vi "svfa_Process FRF (Nx1).vi"(0 "stimulus signal X [EUx]":waveform(dbl), 1 "response signals Y [EUy]":waveform(dbl)[](array[waveform]), 2 "window":T9=1 items=["None"=0, "Hanning"=1, "Hamming"=2, "Blackman-Harris"=3, "Exact Blackman"=4, "Blackman"=5, "Flat Top"=6, "4 Term B-Harris "=7, "7 Term B-Harris"=8, "Low Sidelobe"=9, "Force - Exponential"=10, "Blackman Nuttall"=11, "Triangle"=30, "Bartlett-Hanning"=31, "Bohman"=32, "Parzen"=33, "Welch"=34, "Kaiser"=60, "Dolph-Chebyshev"=61, "Gaussian"=62], 3 "force/exp settings":T8={"force window [%]"=50.0, "exp window [%]"=10.0} {"exp window [%]" min=0.0 max=100.0 format="%.2f"; "force window [%]" min=0.0 max=100.0 format="%.2f"}, 4 "averaging parameters":T11={"averaging mode"=enum."No averaging", "weighting mode"=enum."Linear", "number of averages"=10, "linear mode"=enum."Auto restart"}, 5 "error in (no error)":errorcluster, 7 "processing control":T10(ring), 9 "FRF mode":enum16{"H1", "H2", "H3"}(ring), 11 "spectra info in":T1[](array[typedef]) {"x-axis units" items=["Time (s)"=0, "Frequency-CB (Hz)"=1, "Frequency-CPB (Hz)"=1248, "Frequency-Arbitrary (Hz)"=2357, "Quefrency (s)"=2, "Revolutions (rev)"=3, "Order"=4, "Speed (RPM)"=11, "Speed (rad/s)"=21, "Index"=65535]; "weighting filter" items=["Linear", "A-weighting", "B-weighting", "C-weighting", "ITU-R 468-4", "Dolby", "CCITT", "C-message", "Wb", "Wc", "Wd", "We", "Wf", "Wh", "Wj", "Wk", "Wm", "AES17 20 kHz lowpass", "AES17 40 kHz lowpass", "AES17 20 kHz highpass", "AES17 40 kHz highpass"]; "dB reference [EU]" format="%.2f"; "engineering units" items=["custom..."=0, "V"=1, "A"=21, "C"=30, "pC"=31, "s"=32, "-"=29, "Pa"=2, "N"=20, "g"=3, "m/s^2"=4, "m/s"=5, "m"=6, "mm/s"=12, "mm"=13, "micron/s"=14, "micron"=15, "in/s^2"=7, "in/s"=8, "in"=9, "mil/s"=10, "mil"=11, "rad/s^2"=16, "rad/s"=17, "rad"=18, "deg/s^2"=26, "deg/s"=27, "deg"=28, "RPM"=22, "cycle/s^2"=23, "Hz"=24, "cycle"=25, "strain"=19]; "spectral info"."window" items=["None "=0, "Hanning"=1, "Hamming"=2, "Blackman-Harris"=3, "Exact Blackman"=4, "Blackman"=5, "Flat Top"=6, "4 Term B-Harris "=7, "7 Term B-Harris"=8, "Low Sidelobe"=9, "Force - Exponential"=10, "Gaussian"=62]}) -> (8 "dup stimulus signal X [EUx]":waveform(dbl), 10 "response signals Y [EUy] 2":waveform(dbl)[](array[waveform]), 12 "averages completed":dbl format="%.2f", 13 "processing control":T10(ring), 14 "complex responses [EUy/EUx]":T7(array[cluster]) {"complex spectrum" format="%.2f"; "df" format="%.2f"; "f0" format="%.2f"}, 16 "coherence":cluster{"f0":dbl, "df":dbl, "coherence":dbl[]}[](array[cluster]) {"coherence" format="%.2f"; "df" format="%.2f"; "f0" format="%.2f"}, 17 "averaging done":bool, 18 "spectra info out":T1[](array[typedef]) {"x-axis units" items=["Time (s)"=0, "Frequency-CB (Hz)"=1, "Frequency-CPB (Hz)"=1248, "Frequency-Arbitrary (Hz)"=2357, "Quefrency (s)"=2, "Revolutions (rev)"=3, "Order"=4, "Speed (RPM)"=11, "Speed (rad/s)"=21, "Index"=65535]; "weighting filter" items=["Linear", "A-weighting", "B-weighting", "C-weighting", "ITU-R 468-4", "Dolby", "CCITT", "C-message", "Wb", "Wc", "Wd", "We", "Wf", "Wh", "Wj", "Wk", "Wm", "AES17 20 kHz lowpass", "AES17 40 kHz lowpass", "AES17 20 kHz highpass", "AES17 40 kHz highpass"]; "dB reference [EU]" format="%.2f"; "engineering units" items=["custom..."=0, "V"=1, "A"=21, "C"=30, "pC"=31, "s"=32, "-"=29, "Pa"=2, "N"=20, "g"=3, "m/s^2"=4, "m/s"=5, "m"=6, "mm/s"=12, "mm"=13, "micron/s"=14, "micron"=15, "in/s^2"=7, "in/s"=8, "in"=9, "mil/s"=10, "mil"=11, "rad/s^2"=16, "rad/s"=17, "rad"=18, "deg/s^2"=26, "deg/s"=27, "deg"=28, "RPM"=22, "cycle/s^2"=23, "Hz"=24, "cycle"=25, "strain"=19]; "spectral info"."window" items=["None "=0, "Hanning"=1, "Hamming"=2, "Blackman-Harris"=3, "Exact Blackman"=4, "Blackman"=5, "Flat Top"=6, "4 Term B-Harris "=7, "7 Term B-Harris"=8, "Low Sidelobe"=9, "Force - Exponential"=10, "Gaussian"=62]}, 19 "error out":errorcluster)   [LabVIEW 2017]
uses:
  <vilib>/addons/_NISVFA/_Shared subVIs/Controls/svc_Window [Dual FFT].ctl
  <vilib>/addons/_NISVFA/_Shared subVIs/Controls/svc_Spectrum Info.ctl
  <vilib>/addons/_NISVFA/_Shared subVIs/Controls/svc_X-Axis Units.ctl
  <vilib>/addons/_NISVFA/_Shared subVIs/Controls/svc_Spectrum Type.ctl
  <vilib>/addons/_NISVFA/_Shared subVIs/Controls/svc_Engineering Units Text Ring.ctl
  <vilib>/addons/_NISVFA/_Shared subVIs/Controls/svc_Weighting Filter Text Ring.ctl
  <vilib>/addons/_NISVFA/_Shared subVIs/Controls/svc_Complimentary Spectrum Units.ctl
  <vilib>/addons/_NISVFA/_Shared subVIs/Windowing/svfa_Scaled Time Domain Window (1 Ch).vi
  <vilib>/addons/_NISVFA/_Shared subVIs/Windowing/svfa_Scaled Time Domain Window (N Ch).vi
  <vilib>/addons/_NISVFA/_Shared subVIs/Spectrum Averaging/svfa_Average Array (real).vi
  <vilib>/addons/_NISVFA/_Shared subVIs/Spectrum Averaging/svfa_Average Array (complex).vi
  <vilib>/addons/_NISVFA/_Shared subVIs/Windowing/svfa_Scaled Time Domain Window (Array).vi
  <vilib>/Analysis/4window.llb/Force Window.vi
  <vilib>/Analysis/4window.llb/Force Window (DBL).vi
  <vilib>/Analysis/4window.llb/Exponential Window.vi
  <vilib>/Analysis/4window.llb/Exponential Window (DBL).vi
  <vilib>/Utility/error.llb/Error Cluster From Error Code.vi
  <vilib>/Analysis/0measdsp.llb/Scaled Time Domain Window.vi
  <vilib>/Analysis/0measdsp.llb/Scaled Time Domain Window (DBL).vi
  <vilib>/addons/_NISVFA/_Spectrum Processing/subVIs/svfa_Spectrum Info Window to windowTd Type Def.vi
  <vilib>/addons/_NISVFA/_Shared subVIs/Common/svc_Window Parameters.vi
  <vilib>/addons/_NISVFA/_Shared subVIs/Common/svc_Get Window Info.vi
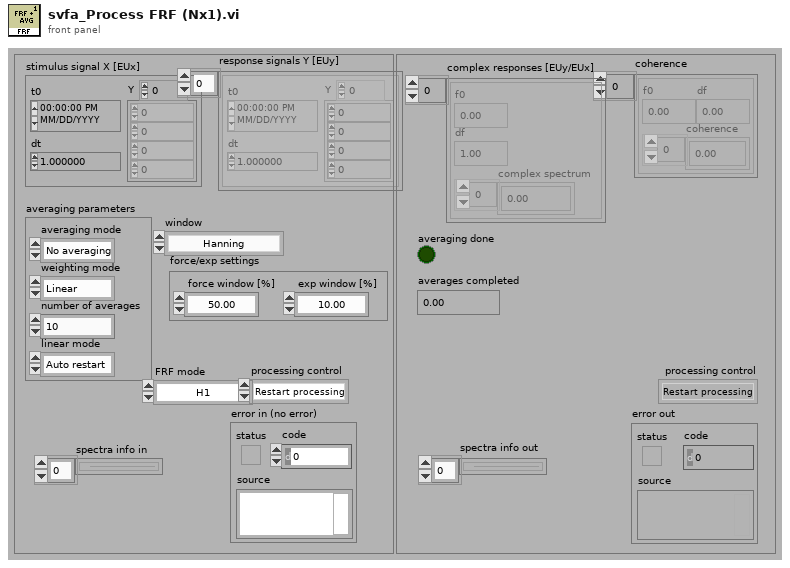
[diagram p1: front panel]
types:
  T1 = typedef "svc_Spectrum Info.ctl" = cluster{"channel name":string, "description":string, "x-axis units":T2, "spectral info":cluster{"spectrum type":T3, "linear/dB":enum16{"linear", "dB"}, "window":u16, "window size":i32, "FFT size":i32}, "engineering units":T4, "custom label":string, "dB reference [EU]":dbl, "peak units":enum16{"rms", "peak", "peak-peak"}, "weighting filter":T5, "spectral density?":bool, "unit label":string, "spectrum skewed?":bool, "complimentary spectrum units":T6}
  T2 = typedef "svc_X-Axis Units.ctl" = u16
  T3 = typedef "svc_Spectrum Type.ctl" = enum16{"FFT Spectrum [complex]", "Amplitude [Magnitude]", "Power [Magnitude^2]", "Cross Spectrum [complex]", "Frequency Response [Complex]"}
  T4 = typedef "svc_Engineering Units Text Ring.ctl" = u16
  T5 = typedef "svc_Weighting Filter Text Ring.ctl" = u16
  T6 = typedef "svc_Complimentary Spectrum Units.ctl" = enum16{"none", "radians", "degrees", "cycles", "imaginary"}
  T7 = cluster{"f0":dbl, "df":dbl, "complex spectrum":cdb[]}[]
  T8 = cluster{"force window [%]":dbl, "exp window [%]":dbl}
  T9 = typedef "svc_Window [Dual FFT].ctl" = u32
  T10 = enum16{"Restart processing", "Continue processing", "Skip processing"}
  T11 = cluster{"averaging mode":enum16{"No averaging", "Vector averaging", "RMS averaging", "Peak hold"}, "weighting mode":enum16{"Linear", "Exponential"}, "number of averages":u32, "linear mode":enum16{"One shot", "Auto restart"}}
  T12 = enum16{"No averaging", "Vector averaging", "RMS averaging", "Peak hold"}
  T13 = cluster{"f0":dbl, "df":dbl, "complex array":cdb[]}
  T14 = cluster{"f0":dbl, "df":dbl, "complex array":cdb[]}[]
  T15 = cluster{"complex spectrum":cluster{"f0":dbl, "df":dbl, "complex spectrum":cdb[]}, "spectrum info":T1}
  T16 = cluster{"f0":dbl, "df":dbl, "complex spectrum":cdb[]}
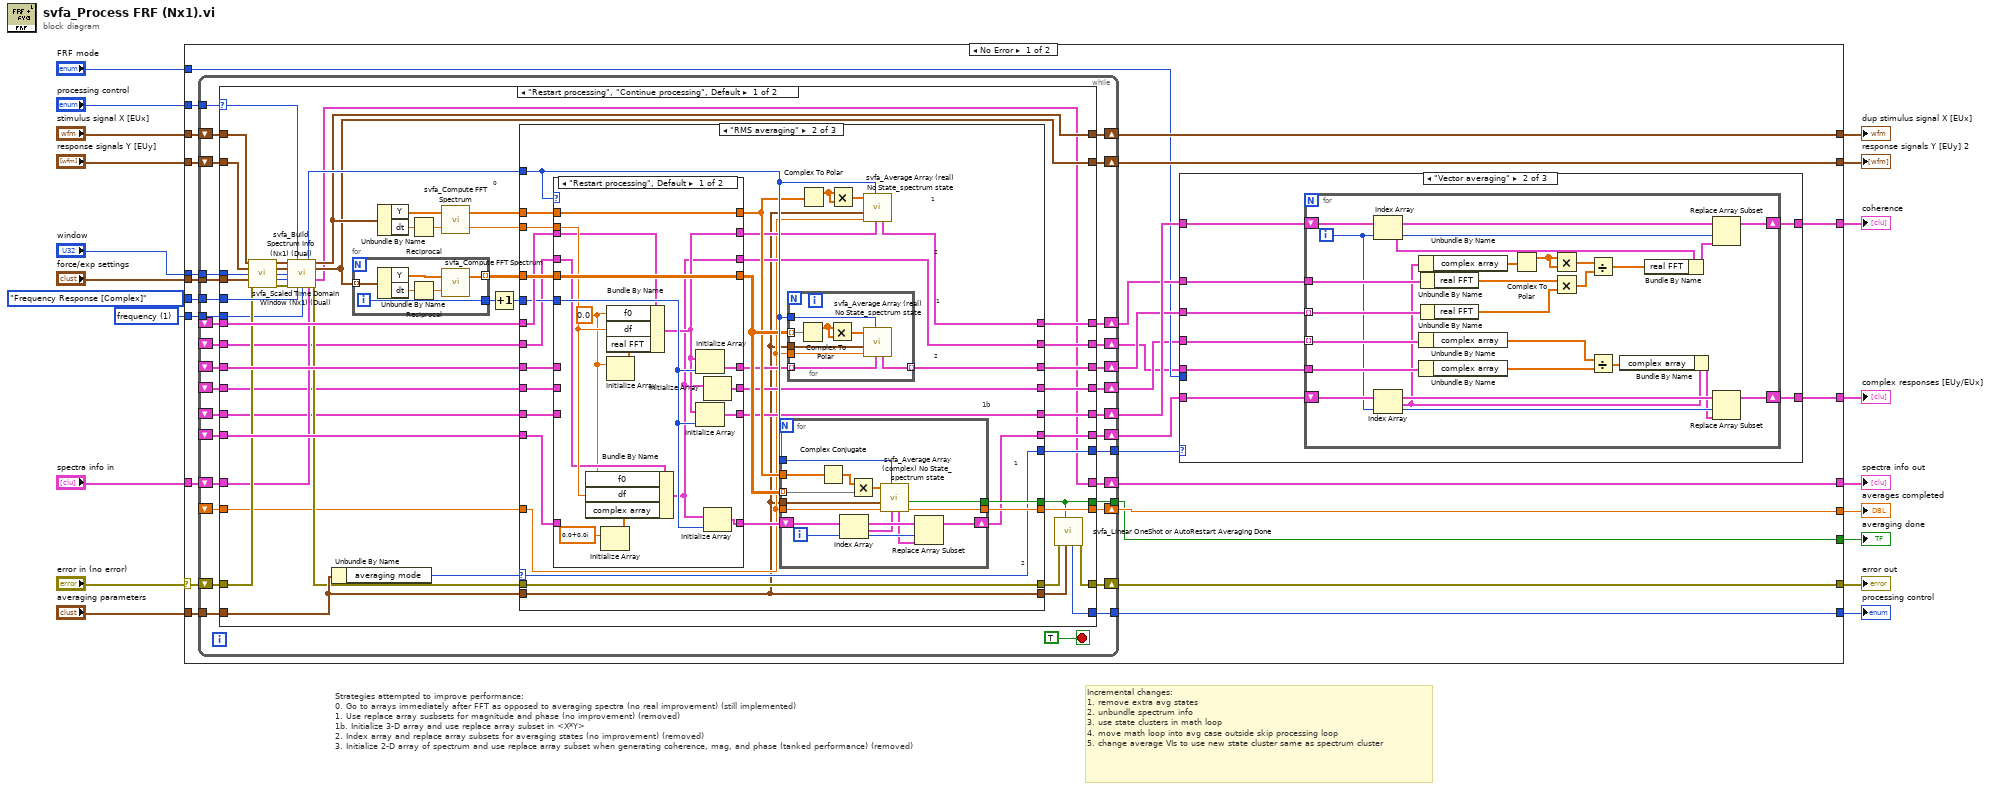
[diagram p0: block diagram]
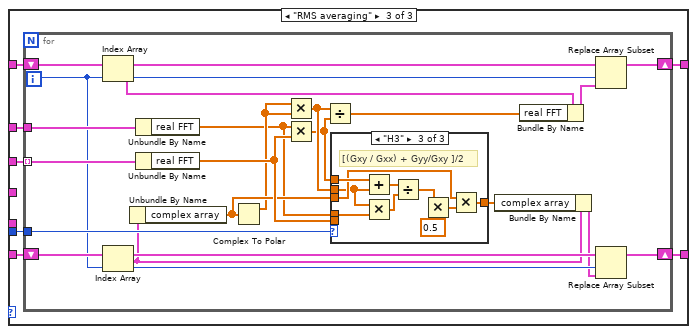
[diagram p3: hidden frame]
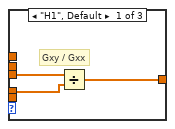
[diagram p4: hidden frame]
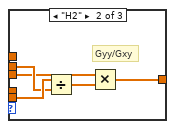
[diagram p5: hidden frame]
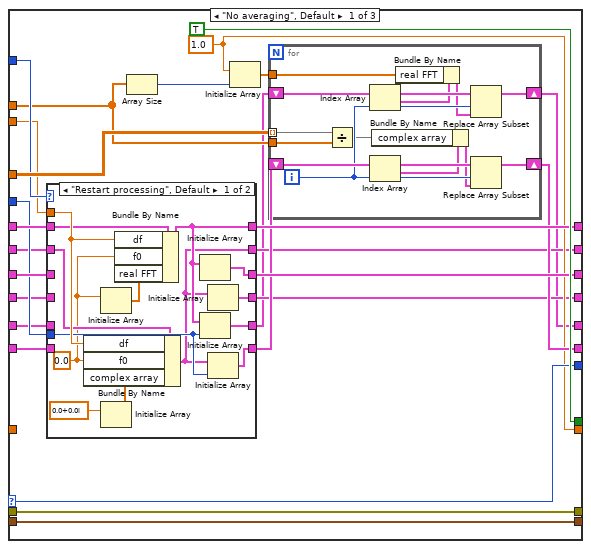
[diagram p6: hidden frame]
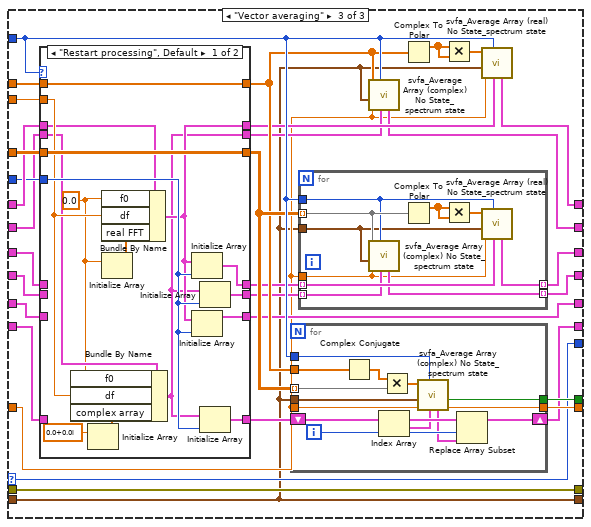
[diagram p9: hidden frame]
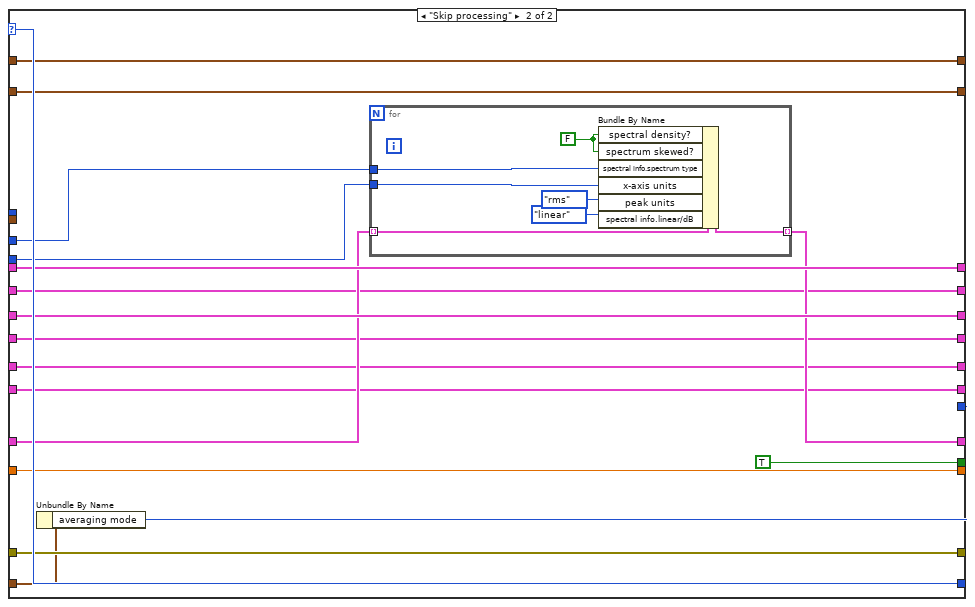
[diagram p11: hidden frame]
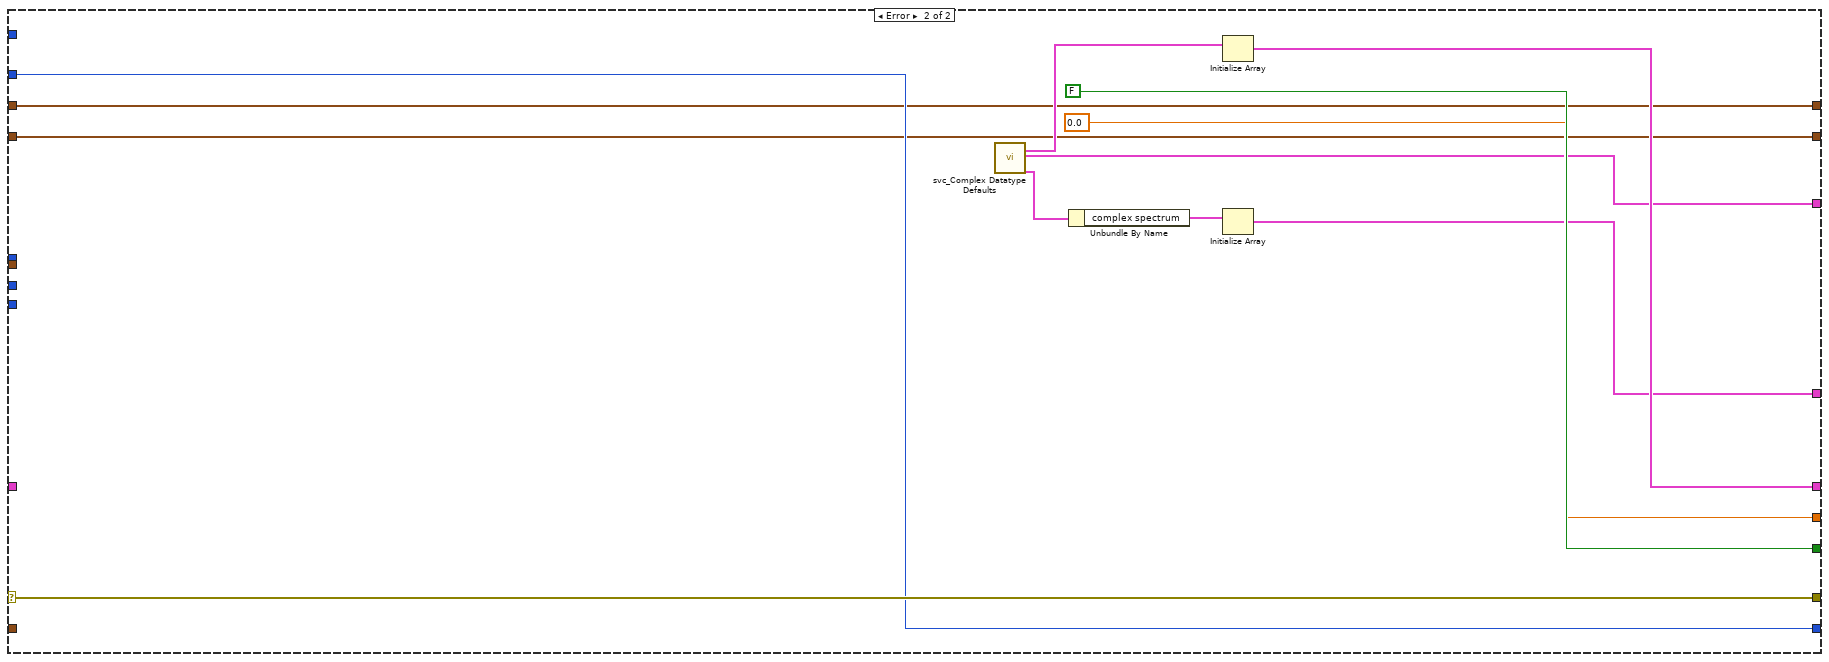
[diagram p12: hidden frame]
diagram:
  w6 = u16 1 items=["time"=0, "frequency"=1, "quefrency"=2, "revolutions"=3, "order"=4, "rpm"=11] ("x-axis units")
  # "Strategies attempted to improve performance:\n0. Go to arrays immediately after FFT as opposed to averaging spectra (no real improvement) (still implemented)\n1. Use replace array susbsets for magnitude and phase (no improvement) (removed)\n1b. Initialize 3-D array and use replace array subset in <X*Y>\n2. Index array and replace array subsets for averaging states (no improvement) (removed)\n3. Initialize 2-D array of spectrum and use replace array subset when generating coherence, mag, and phase (tanked performance) (removed)"
  # "Incremental changes:\n1. remove extra avg states\n2. unbundle spectrum info\n3. use state clusters in math loop\n4. move math loop into avg case outside skip processing loop\n5. change average VIs to use new state cluster same as spectrum cluster"
  n1 = case shown="No Error" "error in (no error)" {
    selector: "error in (no error)" -> [w44 w464]
    tunnel: [w38 w464] -> w20
    tunnel: "averaging parameters" -> [w47 _]
    tunnel: "stimulus signal X [EUx]" -> [w45 w455]
    tunnel: [w32 FALSE ("averaging done")] -> w16
    tunnel: [w46 0.0 ("averages completed")] -> w15
    tunnel: [w22 w456] -> w14
    tunnel: [w23 w453] -> w13
    tunnel: "FRF mode" -> [w26 _]
    tunnel: "processing control" -> [w43 w461]
    tunnel: [w39 w461] -> w10
    tunnel: "response signals Y [EUy]" -> [w42 w454]
    tunnel: "window" -> [w41 _]
    tunnel: "force/exp settings" -> [w40 _]
    tunnel: svc_Spectrum_Type."Frequency Response [Complex]" ("spectrum type") -> [w37 _]
    tunnel: w6 -> [w36 _]
    tunnel: [w35 w459] -> w5
    tunnel: [w34 w455] -> w4
    tunnel: [w33 w454] -> w3
    tunnel: "spectra info in" -> [w21 _]
    frame No Error {
      n2 = while {
        tunnel: [w149] -> w39
        tunnel: w40 -> [w150]
        tunnel: w41 -> [w151]
        tunnel: w43 -> [w146]
        tunnel: [w155] -> w32
        tunnel: w47 -> [w157]
        shift-right: [w145] -> w28
        shift-left: _ -> [w144]
        shift-right: [w127] -> w31
        shift-left: _ -> [w130]
        shift-right: [w143] -> w29
        shift-left: _ -> [w142]
        tunnel: w37 -> [w141]
        tunnel: w36 -> [w140]
        tunnel: [w137] -> w27
        shift-right: [w136] -> w34
        shift-left: w45 -> [w154]
        shift-right: [w135] -> w33
        shift-left: w42 -> [w152]
        shift-right: [w148] -> w38
        shift-left: w44 -> [w153]
        shift-right: [w138] -> w35
        shift-left: w21 -> [w139]
        shift-right: [w129] -> w24
        shift-left: _ -> [w132]
        shift-right: [w128] -> w25
        shift-left: _ -> [w131]
        shift-right: [w134] -> w30
        shift-left: _ -> [w133]
        shift-right: [w156] -> w46
        shift-left: _ -> [w126]
        stop <- TRUE stop-if-true
        n3 = case shown="\"Restart processing\", \"Continue processing\", Default" w146 {
          selector: w146 -> [w158 w445]
          tunnel: w157 -> [w193 w436]
          tunnel: [w205 w432] -> w156
          tunnel: [w204 TRUE ("averaging done")] -> w155
          tunnel: w153 -> [w179 w443]
          tunnel: w152 -> [w200 w433]
          tunnel: w151 -> [w199 _]
          tunnel: w150 -> [w189 _]
          tunnel: [w196 w445] -> w149
          tunnel: [w194 w443] -> w148
          tunnel: w154 -> [w201 w434]
          tunnel: [w188 w437] -> w134
          tunnel: [w187 w442] -> w145
          tunnel: w133 -> [w186 w437]
          tunnel: w144 -> [w185 w442]
          tunnel: [w184 w441] -> w143
          tunnel: w142 -> [w183 w441]
          tunnel: w141 -> [w182 w428]
          tunnel: w140 -> [w176 w438]
          tunnel: w139 -> [w175 w440]
          tunnel: [w162 w439] -> w138
          tunnel: [w174 w435] -> w137
          tunnel: [w171 w434] -> w136
          tunnel: [w170 w433] -> w135
          tunnel: w132 -> [w169 w431]
          tunnel: w131 -> [w168 w430]
          tunnel: w130 -> [w167 w429]
          tunnel: [w166 w431] -> w129
          tunnel: [w165 w430] -> w128
          tunnel: [w164 w429] -> w127
          tunnel: w126 -> [w163 w432]
          frame "Restart processing", "Continue processing", Default {
            # "0"
            n4 = call <vilib>:"svfa_Scaled Time Domain Window (Nx1) (Dual).vi"("stimulus signal X [EUx]"=w201, "response signals Y [EUy]"=w200, "window"=w199, "force and exponential window settings"=w189, "error in (no error)"=w179) -> ("stimulus signal X [EUx]"=w203:waveform(dbl), "response signals Y [EUy]"=w202:waveform(dbl)[], "window"=w198:T9, "window size"=w191:i32, "error out"=w190:errorcluster)  [unwired: 6 in]
            n5 = call <vilib>:"svfa_Build Spectrum Info (Nx1) (Dual).vi"("stimulus signal X [EUx]"=w203, "processing control"=w158, "response signals Y [EUy]"=w202, "window"=w198, "window size"=w191, "error in (no error)"=w190, "spectrum type"=w182, "x-axis units"=w176, "spectrum info in"=w175) -> ("dup processing control"=w195:T10, "dup stimulus signal X [EUx]"=w171:waveform(dbl), "response signals Y [EUy]"=w170:waveform(dbl)[], "spectra info out"=w162:T1[], "error out"=w172:errorcluster)  [unwired: 2 in]
            n6 = Unbundle By Name(w193) -> ("averaging mode"=w206:T12)
            n7 = for {
              tunnel: w170 -> [w212] mode=indexing
              tunnel: [w208] -> w181 mode=indexing
              tunnel: [w207] -> w178
              i -> [w207]
              n8 = Unbundle By Name ("Get Waveform Components")(w212) -> ("Y"=w211:dbl[], "dt"=w210:dbl)
              n9 = Reciprocal(x=w210) -> (1/x=w209:dbl)
              n10 = call <vilib>:"svfa_Compute FFT Spectrum.vi"("sampling frequency [Hz]"=w209, "signal [EU]"=w211) -> ("FFT spectrum [EUrms]"=w208:cdb[])  [unwired: 1 out]
            }
            n11 = Unbundle By Name ("Get Waveform Components")(w171) -> ("Y"=w161:dbl[], "dt"=w160:dbl)
            n12 = Reciprocal(x=w160) -> (1/x=w159:dbl)
            n13 = call <vilib>:"svfa_Compute FFT Spectrum.vi"("sampling frequency [Hz]"=w159, "signal [EU]"=w161) -> ("df [Hz]"=w173:dbl, "FFT spectrum [EUrms]"=w192:cdb[])
            n14 = Increment(x=w178) -> (x+1=w177:i32)
            n15 = case shown="\"RMS averaging\"" w206 {
              selector: w206 -> [w225 w283 w361]
              tunnel: [w236 w282 w360] -> w180
              tunnel: w172 -> [w236 w282 w360]
              tunnel: w193 -> [w237 w274 w350]
              tunnel: [TRUE ("averaging done") w301 w379] -> w204
              tunnel: w195 -> [w234 w299 w377]
              tunnel: [w222 w300 w378] -> w205
              tunnel: [w237 w274 w350] -> w197
              tunnel: w192 -> [w223 w297 w375]
              tunnel: w181 -> [w235 w298 w376]
              tunnel: [w226 w287 w362] -> w188
              tunnel: [w229 w285 w364] -> w187
              tunnel: w186 -> [w231 w291 w370]
              tunnel: w185 -> [w232 w290 w367]
              tunnel: [w230 w286 w365] -> w184
              tunnel: w183 -> [w233 w289 w368]
              tunnel: w173 -> [w224 w284 w363]
              tunnel: w177 -> [w228 w288 w366]
              tunnel: [w225 w283 w361] -> w174
              tunnel: w169 -> [w217 w280 w354]
              tunnel: w168 -> [w219 w278 w353]
              tunnel: w167 -> [w220 w276 w352]
              tunnel: [w218 w281 w358] -> w166
              tunnel: [w216 w279 w356] -> w165
              tunnel: [w214 w277 w355] -> w164
              tunnel: w163 -> [_ w275 w351]
              frame "No averaging", Default {
                w222 = 1.0 ("overwrite value")
                n16 = case shown="\"Restart processing\", Default" w234 {
                  tunnel: [w245 w258] -> w230
                  tunnel: w233 -> [w246 w258]
                  tunnel: [w248 w257] -> w229
                  tunnel: w232 -> [_ w257]
                  tunnel: [w252 w256] -> w227
                  tunnel: w231 -> [_ w256]
                  tunnel: w228 -> [w249 _]
                  tunnel: w224 -> [w251 _]
                  tunnel: w220 -> [_ w253]
                  tunnel: w219 -> [_ w254]
                  tunnel: w217 -> [w244 w255]
                  tunnel: [w243 w255] -> w218
                  tunnel: [w247 w254] -> w216
                  tunnel: [w250 w253] -> w215
                  frame "Restart processing", Default {
                    w242 = 0.0 ("f0")
                    n17 = Initialize Array(w242) -> (w241:dbl[])  [unwired: 1 in]
                    n18 = Initialize Array(cdb 0.0+0.0i ("element")) -> (w239:cdb[])  [unwired: 1 in]
                    n19 = Bundle By Name(cluster=w244, "df"=w251, "f0"=w242, "complex array"=w239) -> (w243:T13)
                    n20 = Bundle By Name(cluster=w246, "df"=w251, "f0"=w242, "real FFT"=w241) -> (w245:cluster{"f0":dbl, "df":dbl, "real FFT":dbl[]})
                    n21 = Initialize Array(w245) -> (w248:cluster{"f0":dbl, "df":dbl, "real FFT":dbl[]}[])  [unwired: 1 in]
                    n22 = Initialize Array(w245, w249) -> (w250:cluster{"f0":dbl, "df":dbl, "real FFT":dbl[]}[])
                    n23 = Initialize Array(w243) -> (w247:T14)  [unwired: 1 in]
                    n24 = Initialize Array(w243, w249) -> (w252:T14)
                  }
                  frame "Continue processing" {
                  }
                }
                n25 = Array Size(array=w223) -> (size(s)=w213:i32)
                n26 = Initialize Array(w222, w213) -> (w221:dbl[])
                n27 = for {
                  tunnel: w221 -> [w269]
                  tunnel: w223 -> [w271]
                  tunnel: w235 -> [w270] mode=indexing
                  shift-right: [w267] -> w226
                  shift-left: w227 -> [w268]
                  shift-right: [w264] -> w214
                  shift-left: w215 -> [w265]
                  i -> [w266]
                  n28 = Divide(x=w270, y=w271) -> (x/y=w263:cdb[])
                  n29 = Index Array(array=w265, index=w266) -> (element=w260:cluster{"f0":dbl, "df":dbl, "real FFT":dbl[]})
                  n30 = Index Array(array=w268, index=w266) -> (element=w261:T13)
                  n31 = Bundle By Name(cluster=w261, "complex array"=w263) -> (w262:T13)
                  n32 = Bundle By Name(cluster=w260, "real FFT"=w269) -> (w259:cluster{"f0":dbl, "df":dbl, "real FFT":dbl[]})
                  n33 = Replace Array Subset(array=w265, new element=w259, index=w266) -> (w264:cluster{"f0":dbl, "df":dbl, "real FFT":dbl[]}[])
                  n34 = Replace Array Subset(array=w268, new element=w262, index=w266) -> (w267:T14)
                }
              }
              frame "RMS averaging" {
                # "1"
                # "1b"
                # "2"
                # "2"
                # "2"
                # "1"
                # "1"
                n35 = case shown="\"Restart processing\", Default" w299 {
                  tunnel: w298 -> [w317 w322]
                  tunnel: w297 -> [w310 w325]
                  tunnel: [w317 w322] -> w296
                  tunnel: [w310 w325] -> w295
                  tunnel: [w316 w324] -> w294
                  tunnel: [w307 w323] -> w293
                  tunnel: [w315 w321] -> w292
                  tunnel: w291 -> [_ w324]
                  tunnel: w289 -> [w308 w323]
                  tunnel: w290 -> [_ w321]
                  tunnel: w288 -> [w314 _]
                  tunnel: w284 -> [w313 _]
                  tunnel: [w302 w320] -> w281
                  tunnel: w280 -> [w306 w320]
                  tunnel: [w312 w319] -> w279
                  tunnel: w278 -> [_ w319]
                  tunnel: [w311 w318] -> w277
                  tunnel: w276 -> [_ w318]
                  frame "Restart processing", Default {
                    w305 = 0.0 ("f0")
                    n36 = Initialize Array(cdb 0.0+0.0i ("element")) -> (w303:cdb[])  [unwired: 1 in]
                    n37 = Bundle By Name(cluster=w306, "f0"=w305, "df"=w313, "complex array"=w303) -> (w302:T13)
                    n38 = Initialize Array(w305) -> (w309:dbl[])  [unwired: 1 in]
                    n39 = Bundle By Name(cluster=w308, "f0"=w305, "df"=w313, "real FFT"=w309) -> (w307:cluster{"f0":dbl, "df":dbl, "real FFT":dbl[]})
                    n40 = Initialize Array(w307, w314) -> (w315:cluster{"f0":dbl, "df":dbl, "real FFT":dbl[]}[])
                    n41 = Initialize Array(w307, w314) -> (w311:cluster{"f0":dbl, "df":dbl, "real FFT":dbl[]}[])
                    n42 = Initialize Array(w302) -> (w312:T14)  [unwired: 1 in]
                    n43 = Initialize Array(w302, w314) -> (w316:T14)
                  }
                  frame "Continue processing", "Skip processing" {
                  }
                }
                n44 = for {
                  tunnel: w295 -> [w339]
                  tunnel: w296 -> [w338] mode=indexing
                  tunnel: w299 -> [w337]
                  tunnel: w274 -> [w336]
                  tunnel: [w335] -> w301
                  tunnel: [w334] -> w300
                  shift-right: [w332] -> w287
                  shift-left: w294 -> [w333]
                  tunnel: w275 -> [w330]
                  i -> [w331]
                  n45 = Complex Conjugate(1:w339) -> (0:w326:cdb[])
                  n46 = Index Array(array=w333, index=w331) -> (element=w327:T13)
                  n47 = Multiply(x=w326, y=w338) -> (x*y=w329:cdb[])
                  n48 = call <vilib>:"svfa_Average Array (complex) No State_spectrum state.vi"("previous avg complex spectrum"=w327, "processing control"=w337, "averages completed in"=w330, "averaging parameters"=w336, "array"=w329) -> ("averages completed out"=w334:dbl, "averaging done"=w335:bool, "avg complex spectrum"=w328:T13)  [unwired: 4 in]
                  n49 = Replace Array Subset(array=w333, new element=w328, index=w331) -> (w332:T14)
                }
                n50 = for {
                  tunnel: w296 -> [w344] mode=indexing
                  tunnel: w299 -> [w347]
                  tunnel: w274 -> [w346]
                  tunnel: w292 -> [w342] mode=indexing
                  tunnel: [w341] -> w285 mode=indexing
                  tunnel: w275 -> [w340]
                  n51 = Complex To Polar(r * e^(i*theta)=w344) -> (r=w345:dbl[])  [unwired: 1 out]
                  n52 = Multiply(x=w345, y=w345) -> (x*y=w343:dbl[])
                  n53 = call <vilib>:"svfa_Average Array (real) No State_spectrum state.vi"("previous avg real spectrum"=w342, "processing control"=w347, "averages completed"=w340, "averaging parameters"=w346, "array"=w343) -> ("new avg real spectrum"=w341:cluster{"f0":dbl, "df":dbl, "real FFT":dbl[]})  [unwired: 4 in, 2 out]
                }
                n54 = Complex To Polar(r * e^(i*theta)=w295) -> (r=w273:dbl[])  [unwired: 1 out]
                n55 = Multiply(x=w273, y=w273) -> (x*y=w272:dbl[])
                n56 = call <vilib>:"svfa_Average Array (real) No State_spectrum state.vi"("previous avg real spectrum"=w293, "processing control"=w299, "averages completed"=w275, "averaging parameters"=w274, "array"=w272) -> ("new avg real spectrum"=w286:cluster{"f0":dbl, "df":dbl, "real FFT":dbl[]})  [unwired: 4 in, 2 out]
              }
              frame "Vector averaging" {
                n57 = case shown="\"Restart processing\", Default" w377 {
                  tunnel: w376 -> [w395 w403]
                  tunnel: w375 -> [w388 w402]
                  tunnel: [w395 w403] -> w374
                  tunnel: [w388 w402] -> w373
                  tunnel: [w394 w401] -> w372
                  tunnel: [w386 w400] -> w371
                  tunnel: w370 -> [_ w401]
                  tunnel: w368 -> [w387 w400]
                  tunnel: [w393 w399] -> w369
                  tunnel: w367 -> [_ w399]
                  tunnel: w366 -> [w392 _]
                  tunnel: w363 -> [w389 _]
                  tunnel: [w384 w398] -> w359
                  tunnel: [w391 w397] -> w357
                  tunnel: [w390 w396] -> w355
                  tunnel: w354 -> [w385 w398]
                  tunnel: w353 -> [_ w397]
                  tunnel: w352 -> [_ w396]
                  frame "Restart processing", Default {
                    w382 = 0.0 ("f0")
                    n58 = Initialize Array(cdb 0.0+0.0i ("f0")) -> (w380:cdb[])  [unwired: 1 in]
                    n59 = Bundle By Name(cluster=w385, "f0"=w382, "df"=w389, "complex array"=w380) -> (w384:T13)
                    n60 = Initialize Array(w382) -> (w383:dbl[])  [unwired: 1 in]
                    n61 = Bundle By Name(cluster=w387, "f0"=w382, "df"=w389, "real FFT"=w383) -> (w386:cluster{"f0":dbl, "df":dbl, "real FFT":dbl[]})
                    n62 = Initialize Array(w386, w392) -> (w393:cluster{"f0":dbl, "df":dbl, "real FFT":dbl[]}[])
                    n63 = Initialize Array(w386, w392) -> (w390:cluster{"f0":dbl, "df":dbl, "real FFT":dbl[]}[])
                    n64 = Initialize Array(w384, w392) -> (w391:T14)
                    n65 = Initialize Array(w384, w392) -> (w394:T14)
                  }
                  frame "Continue processing", "Skip processing" {
                  }
                }
                n66 = for {
                  tunnel: w373 -> [w417]
                  tunnel: w374 -> [w416] mode=indexing
                  tunnel: w377 -> [w415]
                  tunnel: w350 -> [w414]
                  tunnel: [w413] -> w379
                  tunnel: [w412] -> w378
                  shift-right: [w410] -> w362
                  shift-left: w372 -> [w411]
                  tunnel: w351 -> [w408]
                  i -> [w409]
                  n67 = Complex Conjugate(1:w417) -> (0:w407:cdb[])
                  n68 = Index Array(array=w411, index=w409) -> (element=w404:T13)
                  n69 = Multiply(x=w407, y=w416) -> (x*y=w406:cdb[])
                  n70 = call <vilib>:"svfa_Average Array (complex) No State_spectrum state.vi"("previous avg complex spectrum"=w404, "processing control"=w415, "averages completed in"=w408, "averaging parameters"=w414, "array"=w406) -> ("averages completed out"=w412:dbl, "averaging done"=w413:bool, "avg complex spectrum"=w405:T13)  [unwired: 4 in]
                  n71 = Replace Array Subset(array=w411, new element=w405, index=w409) -> (w410:T14)
                }
                n72 = for {
                  tunnel: w374 -> [w427] mode=indexing
                  tunnel: w377 -> [w425]
                  tunnel: w350 -> [w418]
                  tunnel: [w426] -> w364 mode=indexing
                  tunnel: w369 -> [w422] mode=indexing
                  tunnel: w357 -> [w421] mode=indexing
                  tunnel: [w420] -> w356 mode=indexing
                  tunnel: w351 -> [w419]
                  n73 = call <vilib>:"svfa_Average Array (complex) No State_spectrum state.vi"("previous avg complex spectrum"=w421, "processing control"=w425, "averages completed in"=w419, "averaging parameters"=w418, "array"=w427) -> ("avg complex spectrum"=w420:T13)  [unwired: 4 in, 2 out]
                  n74 = Complex To Polar(r * e^(i*theta)=w427) -> (r=w424:dbl[])  [unwired: 1 out]
                  n75 = Multiply(x=w424, y=w424) -> (x*y=w423:dbl[])
                  n76 = call <vilib>:"svfa_Average Array (real) No State_spectrum state.vi"("previous avg real spectrum"=w422, "processing control"=w425, "averages completed"=w419, "averaging parameters"=w418, "array"=w423) -> ("new avg real spectrum"=w426:cluster{"f0":dbl, "df":dbl, "real FFT":dbl[]})  [unwired: 4 in, 2 out]
                }
                n77 = call <vilib>:"svfa_Average Array (complex) No State_spectrum state.vi"("previous avg complex spectrum"=w359, "processing control"=w377, "averages completed in"=w351, "averaging parameters"=w350, "array"=w373) -> ("avg complex spectrum"=w358:T13)  [unwired: 4 in, 2 out]
                n78 = Complex To Polar(r * e^(i*theta)=w373) -> (r=w349:dbl[])  [unwired: 1 out]
                n79 = Multiply(x=w349, y=w349) -> (x*y=w348:dbl[])
                n80 = call <vilib>:"svfa_Average Array (real) No State_spectrum state.vi"("previous avg real spectrum"=w371, "processing control"=w377, "averages completed"=w351, "averaging parameters"=w350, "array"=w348) -> ("new avg real spectrum"=w365:cluster{"f0":dbl, "df":dbl, "real FFT":dbl[]})  [unwired: 4 in, 2 out]
              }
            }
            n81 = call <vilib>:"svfa_Linear OneShot or AutoRestart Averaging Done.vi"("averaging parameters"=w197, "averaging done"=w204, "error in (no error)"=w180) -> ("error out"=w194:errorcluster, "processing control"=w196:T10)  [unwired: 7 in]
          }
          frame "Skip processing" {
            n82 = Unbundle By Name(w436) -> ("averaging mode"=w435:T12)
            n83 = for {
              tunnel: w440 -> [w452] mode=indexing
              tunnel: [w451] -> w439 mode=indexing
              tunnel: w428 -> [w450]
              tunnel: w438 -> [w449]
              w447 = FALSE ("spectral density?")
              n84 = Bundle By Name(cluster=w452, "spectral density?"=w447, "spectrum skewed?"=w447, "spectral info.spectrum type"=w450, "x-axis units"=w449, "peak units"=enum16{"rms", "peak", "peak-peak"}."rms", "spectral info.linear/dB"=enum16{"linear", "dB"}."linear") -> (w451:T1)
            }
          }
        }
      }
      n85 = case shown="\"Vector averaging\"" w27 {
        tunnel: w30 -> [w48 w57 w85]
        tunnel: w28 -> [_ w56 w86]
        tunnel: w29 -> [_ w55 w87]
        tunnel: [w49 w51 w83] -> w23
        tunnel: [w48 w50 w84] -> w22
        tunnel: w26 -> [_ _ w82]
        tunnel: w31 -> [w49 w52 w81]
        tunnel: w24 -> [_ w54 _]
        tunnel: w25 -> [_ w53 _]
        frame "No averaging", Default {
        }
        frame "Vector averaging" {
          n86 = for {
            tunnel: w55 -> [w80]
            tunnel: w56 -> [w79] mode=indexing
            tunnel: w53 -> [w77] mode=indexing
            tunnel: w54 -> [w76]
            shift-right: [w73] -> w51
            shift-left: w52 -> [w75]
            shift-right: [w72] -> w50
            shift-left: w57 -> [w78]
            i -> [w74]
            n87 = Index Array(array=w75, index=w74) -> (element=w66:cluster{"f0":dbl, "df":dbl, "real FFT":dbl[]})
            n88 = Index Array(array=w78, index=w74) -> (element=w62:T13)
            n89 = Unbundle By Name(w62) -> ("complex array"=w68:cdb[])
            n90 = Unbundle By Name(w77) -> ("complex array"=w67:cdb[])
            n91 = Unbundle By Name(w76) -> ("complex array"=w58:cdb[])
            n92 = Unbundle By Name(w80) -> ("real FFT"=w59:dbl[])
            n93 = Unbundle By Name(w79) -> ("real FFT"=w69:dbl[])
            n94 = Complex To Polar(r * e^(i*theta)=w68) -> (r=w60:dbl[])  [unwired: 1 out]
            n95 = Multiply(x=w60, y=w60) -> (x*y=w71:dbl[])
            n96 = Multiply(x=w59, y=w69) -> (x*y=w70:dbl[])
            n97 = Divide(x=w71, y=w70) -> (x/y=w64:dbl[])
            n98 = Divide(x=w67, y=w58) -> (x/y=w61:cdb[])
            n99 = Bundle By Name(cluster=w62, "complex array"=w61) -> (w63:T13)
            n100 = Bundle By Name(cluster=w66, "real FFT"=w64) -> (w65:cluster{"f0":dbl, "df":dbl, "real FFT":dbl[]})
            n101 = Replace Array Subset(array=w75, new element=w65, index=w74) -> (w73:cluster{"f0":dbl, "df":dbl, "real FFT":dbl[]}[])
            n102 = Replace Array Subset(array=w78, new element=w63, index=w74) -> (w72:T14)
          }
        }
        frame "RMS averaging" {
          n103 = for {
            tunnel: w87 -> [w104]
            tunnel: w86 -> [w103] mode=indexing
            tunnel: w82 -> [w102]
            shift-right: [w107] -> w83
            shift-left: w81 -> [w101]
            shift-right: [w106] -> w84
            shift-left: w85 -> [w105]
            i -> [w100]
            n104 = Index Array(array=w101, index=w100) -> (element=w98:cluster{"f0":dbl, "df":dbl, "real FFT":dbl[]})
            n105 = Index Array(array=w105, index=w100) -> (element=w94:T13)
            n106 = Unbundle By Name(w94) -> ("complex array"=w93:cdb[])
            n107 = Unbundle By Name(w104) -> ("real FFT"=w89:dbl[])
            n108 = Unbundle By Name(w103) -> ("real FFT"=w99:dbl[])
            n109 = Complex To Polar(r * e^(i*theta)=w93) -> (r=w90:dbl[])  [unwired: 1 out]
            n110 = Multiply(x=w90, y=w90) -> (x*y=w91:dbl[])
            n111 = Multiply(x=w89, y=w99) -> (x*y=w88:dbl[])
            n112 = Divide(x=w91, y=w88) -> (x/y=w97:dbl[])
            n113 = case shown="\"H3\"" w102 {
              tunnel: [w110 w111 w123] -> w92
              tunnel: w89 -> [w109 _ w119]
              tunnel: w99 -> [_ w115 _]
              tunnel: w93 -> [w108 w112 w117]
              tunnel: w91 -> [_ w114 w116]
              tunnel: w88 -> [_ _ w122]
              frame "H1", Default {
                # "Gxy / Gxx"
                n114 = Divide(x=w108, y=w109) -> (x/y=w110:cdb[])
              }
              frame "H2" {
                # "Gyy/Gxy"
                n115 = Divide(x=w115, y=w114) -> (x/y=w113:dbl[])
                n116 = Multiply(x=w112, y=w113) -> (x*y=w111:cdb[])
              }
              frame "H3" {
                # "[(Gxy / Gxx) + Gyy/Gxy ]/2"
                n117 = Add(x=w122, y=w116) -> (x+y=w121:dbl[])
                n118 = Multiply(x=w116, y=w119) -> (x*y=w118:dbl[])
                n119 = Divide(x=w121, y=w118) -> (x/y=w120:dbl[])
                n120 = Multiply(x=w120, y=0.5) -> (x*y=w124:dbl[])
                n121 = Multiply(x=w117, y=w124) -> (x*y=w123:cdb[])
              }
            }
            n122 = Bundle By Name(cluster=w94, "complex array"=w92) -> (w95:T13)
            n123 = Bundle By Name(cluster=w98, "real FFT"=w97) -> (w96:cluster{"f0":dbl, "df":dbl, "real FFT":dbl[]})
            n124 = Replace Array Subset(array=w101, new element=w96, index=w100) -> (w107:cluster{"f0":dbl, "df":dbl, "real FFT":dbl[]}[])
            n125 = Replace Array Subset(array=w105, new element=w95, index=w100) -> (w106:T14)
          }
        }
      }
    }
    frame Error {
      n126 = call <vilib>:"svc_Complex Datatype Defaults.vi"() -> ("dead spectrum info"=w460:T1, "empty array of spectra"=w453:cluster{"f0":dbl, "df":dbl, "magnitude":dbl[]}[], "complex spectrum"=w458:T15)  [unwired: 11 in, 6 out]
      n127 = Unbundle By Name(w458) -> ("complex spectrum"=w457:T16)
      n128 = Initialize Array(w460) -> (w459:T1[])  [unwired: 1 in]
      n129 = Initialize Array(w457) -> (w456:T7)  [unwired: 1 in]
    }
  }
  "error out" <- w20
  "averages completed" <- w15
  "averaging done" <- w16
  "complex responses [EUy/EUx]" <- w14
  "coherence" <- w13
  "processing control" <- w10
  "spectra info out" <- w5
  "dup stimulus signal X [EUx]" <- w4
  "response signals Y [EUy] 2" <- w3
